vi "String suchen AK.vi"(9 "gesucht":string="NO2 High 191C (2of2)", 11 "Namen":string[](array[string])=["XXX", "NO", "NO2", "NOX"]) -> (1 "Index":i32, 3 "Gefunden?":bool)   [LabVIEW 2020, in "AK-Schnittstelle.lvlib"]
uses:
  AK-Schnittstelle.lvlib
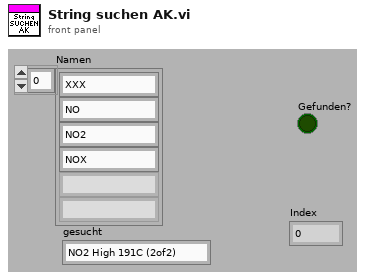
[diagram p1: front panel]
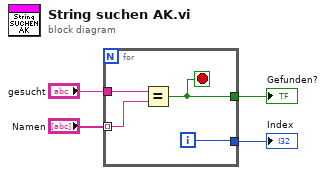
[diagram p0: block diagram]
diagram:
  n1 = for {
    tunnel: "gesucht" -> [w7]
    tunnel: "Namen" -> [w6] mode=indexing
    tunnel: [w5] -> w3
    tunnel: [w8] -> w4
    i -> [w8]
    stop <- w5 stop-if-true
    n2 = Equal?(x=w7, y=w6) -> (x = y?=w5:bool)
  }
  "Index" <- w4
  "Gefunden?" <- w3
